vi "Keithley 622x Error.vi"(8 "error in":errorcluster, 11 "VISA resource name":refnum<visa-resource-name>) -> (0 "error out":errorcluster, 1 "Error text":string, 2 "Error code":i32, 3 "VISA resource name out":refnum<visa-resource-name>, 4 "status byte":u16, 5 "Err buffer":string)   [LabVIEW 2021]
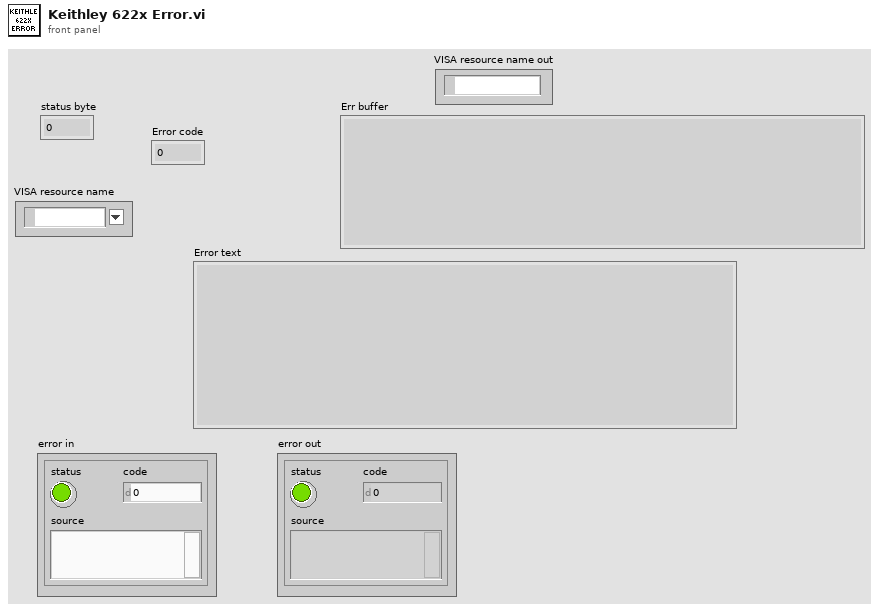
[diagram p1: front panel]
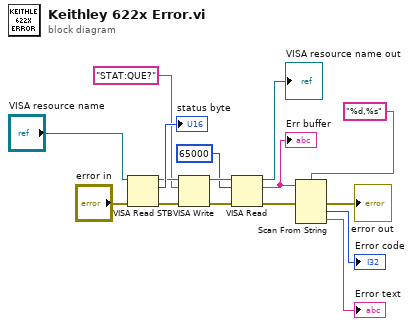
[diagram p0: block diagram]
diagram:
  n1 = VISA Read STB(8:"error in", 11:"VISA resource name") -> (0:w12:errorcluster, 2:→"status byte":u16, 3:w11:refnum<visa-resource-name>)
  n2 = VISA Write(VISA resource name=w11, write buffer="STAT:QUE?", error in (no error)=w12) -> (VISA resource name out=w15:refnum<visa-resource-name>, error out=w14:errorcluster)  [unwired: 1 out]
  n3 = VISA Read(VISA resource name=w15, byte count=u32 65000, error in (no error)=w14) -> (VISA resource name out=→"VISA resource name out":refnum<visa-resource-name>, read buffer=w2:string, error out=w5:errorcluster)  [unwired: 1 out]
  "Err buffer" <- w2
  n4 = Scan From String(format string="%d,%s", input string=w2, error in=w5) -> (error out=→"error out":errorcluster, output 1=→"Error code":i32, output 2=→"Error text":string)  [unwired: 3 in, 2 out]
